vi "函数类型2测试.vi"() -> ()   [LabVIEW 2010]
panel:
  in  "加载配置文件":u16(ring) items=["123.xls", "12333.xls", "1234.xls", "12345.xls", "123666.xls", "12368966.xls"]
  in  "btn_取消":bool
  in  "btn_开始测试":bool
  out "light_32":bool
  out "light_31":bool
  out "light_30":bool
  out "light_29":bool
  out "light_28":bool
  out "light_27":bool
  out "light_26":bool
  out "light_25":bool
  out "light_24":bool
  out "light_23":bool
  out "light_22":bool
  out "light_21":bool
  out "light_20":bool
  out "light_19":bool
  out "light_18":bool
  out "light_17":bool
  out "light_16":bool
  out "light_15":bool
  out "light_14":bool
  out "light_13":bool
  out "light_12":bool
  out "light_11":bool
  out "light_10":bool
  out "light_9":bool
  out "light_8":bool
  out "light_7":bool
  out "light_6":bool
  out "light_5":bool
  out "light_4":bool
  out "light_3":bool
  out "light_2":bool
  out "light_1":bool
  in  "跳变值 2":dbl[](array[numeric])
  in  "跳变值 1":dbl[](array[numeric])
  out "Analog_back":string[][](table) caption="表格"
  in  "Analog_IN":string[][](table) caption="表格"
  # "反馈电平状态"
  # "模拟量输入值（V）"
  # "加载配置文件："
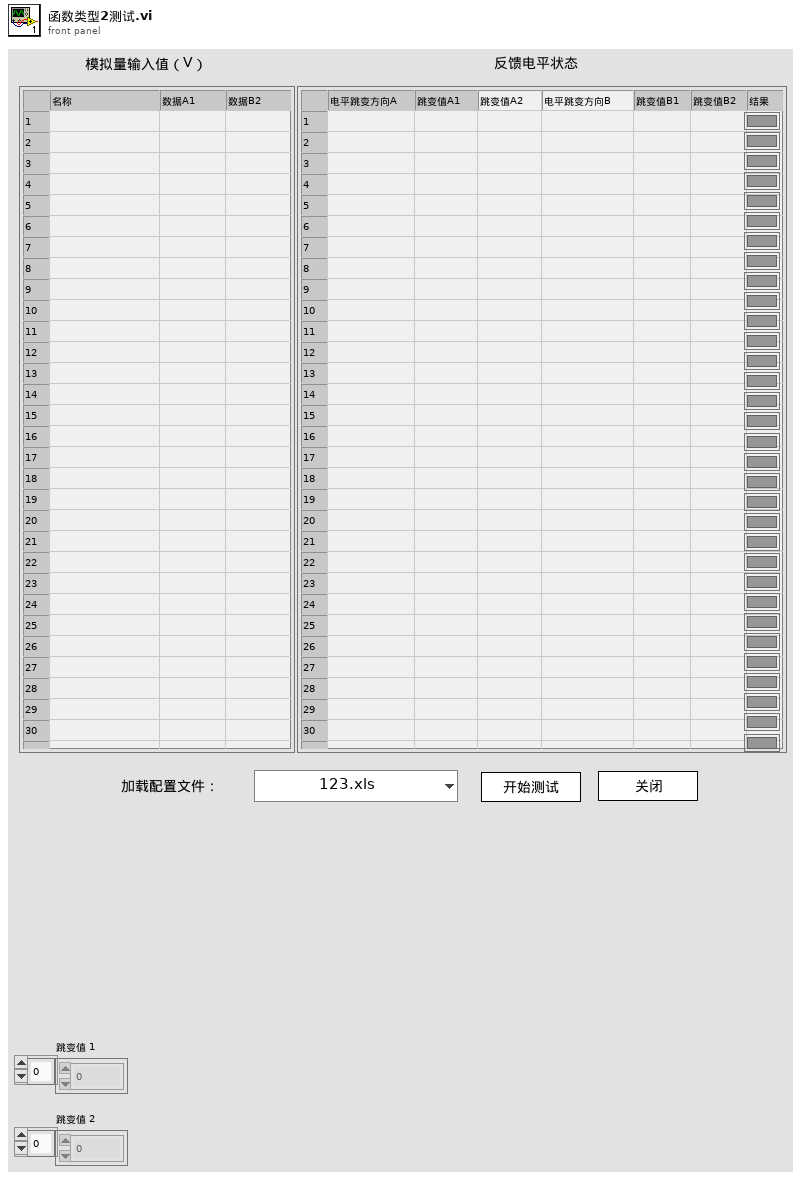
[diagram p1: front panel]
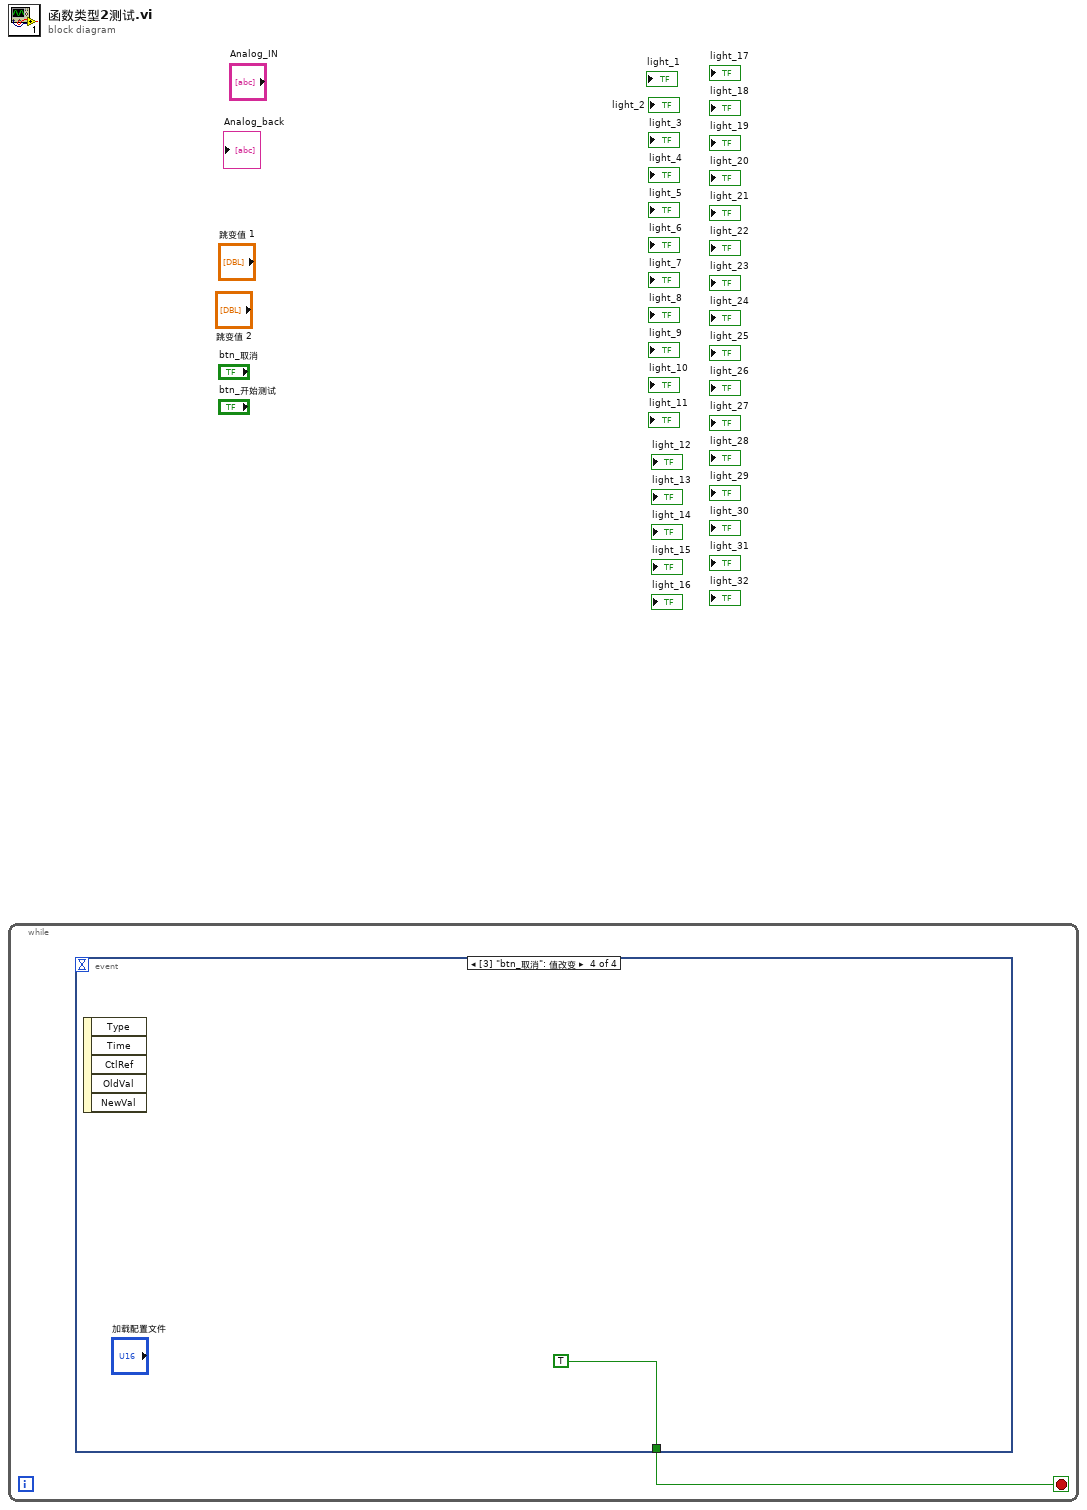
[diagram p0: block diagram]
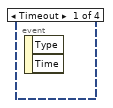
[diagram p2: hidden frame]
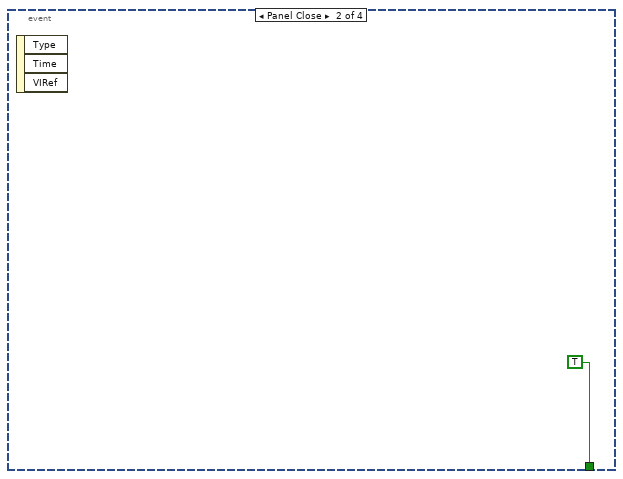
[diagram p3: hidden frame]
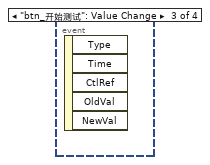
[diagram p4: hidden frame]
diagram:
  n1 = while {
    stop <- w1 stop-if-true
    n2 = event shown="[3] \"btn_取消\": 值改变" {
      selector: _ -> [_ _ _ _]
      dyn-events: _ -> [_ _ _ _]
      timeout: _ -> [_ _ _ _]
      tunnel: [_ TRUE _ TRUE] -> w1
      event Timeout {
        n3 = event-data() -> ()  [unwired: 1 in, 2 out]
      }
      event Panel Close {
        n4 = event-data() -> ()  [unwired: 1 in, 3 out]
      }
      event "btn_开始测试": Value Change {
        n5 = event-data() -> ()  [unwired: 1 in, 5 out]
      }
      event "btn_取消": Value Change {
        n6 = event-data() -> ()  [unwired: 1 in, 5 out]
      }
    }
  }
